vi "Scripting Tests.vi"   [LabVIEW 2018]
uses:
  <vilib>/addons/_JKI Toolkits/Caraya/classes/Test Suite/Define Test Suite (Default).vi
  <vilib>/addons/_JKI Toolkits/Caraya/classes/Test Suite/Test Suite.lvclass
types:
  T1 = enum32{"Invalid", "Standard", "Closed", "Hidden", "Minimized", "Maximized"}
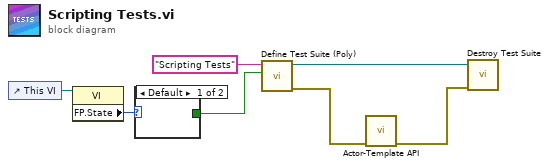
[diagram p0: block diagram]
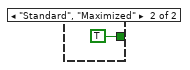
[diagram p2: hidden frame]
diagram:
  n1 = control-ref of="This VI"() -> (w3:refnum<vi>)
  n2 = property class="VI"(reference=w3) -> ("FP.State"=w2:T1)  [unwired: 1 in, 2 out]
  n3 = case shown="Default" w2 {
    tunnel: [_ TRUE] -> w1
    frame Default {
    }
    frame "Standard", "Maximized" {
    }
  }
  n4 = call-poly <vilib>:"Define Test Suite (Poly).vi"("Interactive"=w1, "Label (VI Title)"="Scripting Tests") -> ("error out"=w7:errorcluster, "Test Suite"=w5:refnum<class "Test Suite.lvclass">)  [unwired: 8 in]
  n5 = call "Actor-Template API.vi"("error in (no error)"=w7) -> ("error out"=w4:errorcluster)  [unwired: 10 in]
  n6 = call-dynamic "Destroy Test Suite.vi"("error in (no error)"=w4, "Test Suite in"=w5) -> ()  [unwired: 9 in, 1 out]
